vi "Write Product.vi"(8 "error in (no error)":errorcluster, 10 "Product":refnum<class "Product.lvclass">, 11 "Creator in":refnum<class "Creator.lvclass">) -> (0 "error out":errorcluster, 3 "Creator out":refnum<class "Creator.lvclass">)   [LabVIEW 2020, in "FactoryMethod.lvlib" / "Creator.lvclass"]
uses:
  Creator.lvclass
  Product/Product.lvclass
  Creator.lvclass/Creator.ctl
  TypeDef/privateDataDVR.ctl
  TypeDef/privateData.ctl
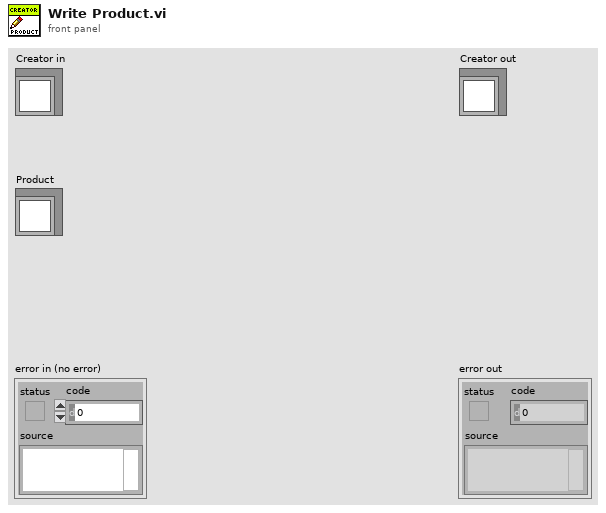
[diagram p1: front panel]
types:
  T1 = typedef "FactoryMethod.lvlib/Creator.lvclass/privateDataDVR.ctl" = refnum<data-value>
  T2 = typedef "FactoryMethod.lvlib/Creator.lvclass/privateData.ctl" = cluster{"Product":refnum<class "Product.lvclass">}
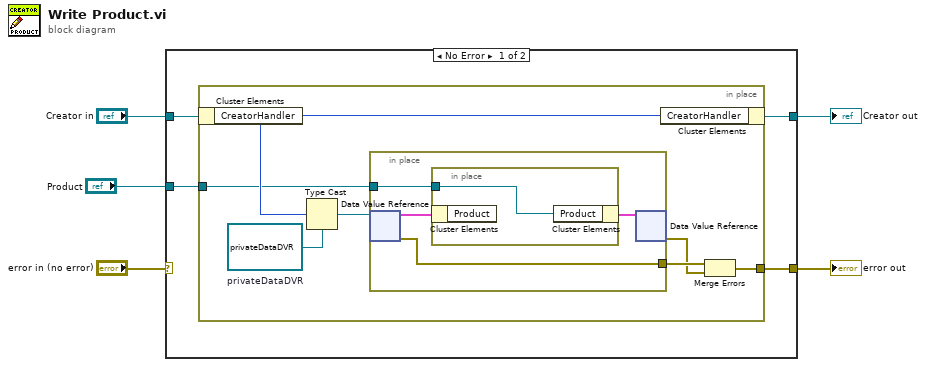
[diagram p0: block diagram]
diagram:
  n1 = case shown="No Error" "error in (no error)" {
    selector: "error in (no error)" -> [_ w23]
    tunnel: [w9 w23] -> w4
    tunnel: [w7 w22] -> w2
    tunnel: "Creator in" -> [w8 w22]
    tunnel: "Product" -> [w6 _]
    frame No Error {
      n2 = in-place {
        in-place-border: [w10] -> w9
        in-place-border: w6 -> [w13]
        w16 = T1 refnum  # privateDataDVR
        n3 = in-place-cluster #1(w8) -> ("CreatorHandler"=w14:u32)
        n4 = Type Cast(type=w16, x=w14) -> (*(type *) &x=w15:T1)
        n5 = in-place {
          in-place-border: [w19] -> w12
          in-place-border: w13 -> [w18]
          n6 = in-place-dvr #2(w15) -> (w20:T2, w19:errorcluster)
          n7 = in-place {
            in-place-border: w18 -> [w21]
            n8 = in-place-cluster #3(w20) -> ()  [unwired: 1 out]
            n9 = in-place-cluster #3("Product"=w21) -> (w17:T2)
          }
          n10 = in-place-dvr #2(w17) -> (w11:errorcluster)  [unwired: 1 out]
        }
        n11 = in-place-cluster #1("CreatorHandler"=w14) -> (w7:refnum<class "Creator.lvclass">)
        n12 = Merge Errors(w12, w11) -> (w10:errorcluster)
      }
    }
    frame Error {
    }
  }
  "error out" <- w4
  "Creator out" <- w2
